vi "Nodos_de_Propiedad_3.vi"() -> ()   [LabVIEW 2016]
panel:
  in  "stop":bool
  out "Boolean":bool
  out "fecha":string
  out "no.muestreo":dbl
  in  "limite superior":dbl
  in  "limite inferior":dbl
  in  "muestras":dbl
  out "temperatura":cluster{dbl, "limite superior":dbl}(graph)
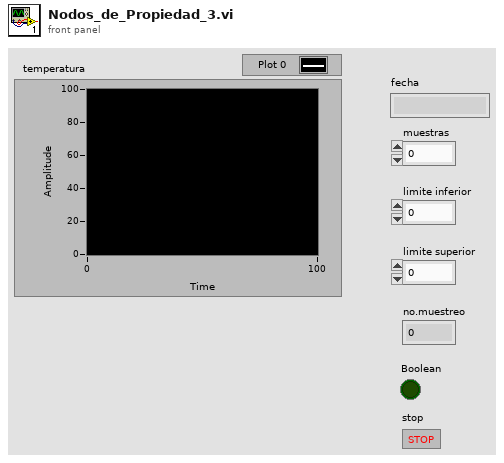
[diagram p1: front panel]
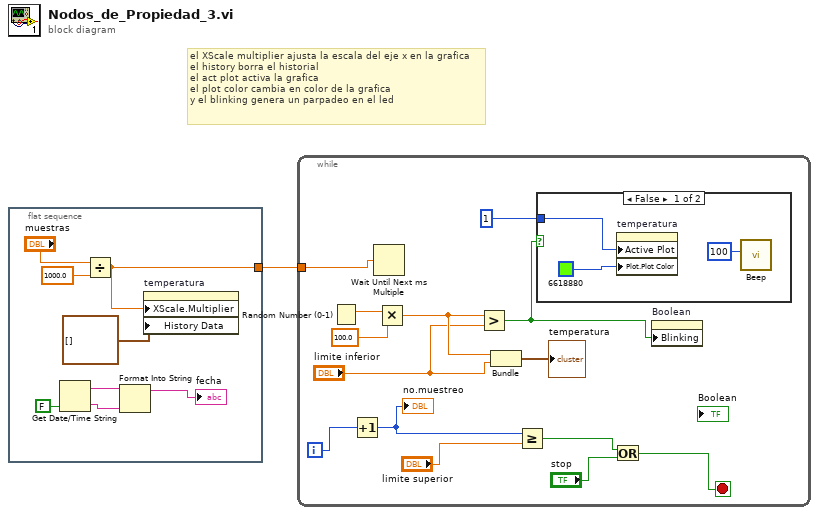
[diagram p0: block diagram]
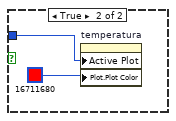
[diagram p2: hidden frame]
diagram:
  # "el XScale multiplier ajusta la escala del eje x en la grafica\nel history borra el historial\nel act plot activa la grafica \nel plot color cambia en color de la grafica\ny el blinking genera un parpadeo en el led"
  n1 = flat-sequence {
    tunnel: [w3] -> w1
    frame #0 {
      n2 = Get Date/Time String(want seconds? (F)=FALSE) -> (date string=w5:string, time string=w6:string)  [unwired: 2 in]
      n3 = Divide(x="muestras", y=1000.0) -> (x/y=w3:dbl)
      n4 = Format Into String(initial string=w5, w6) -> (resulting string=→"fecha":string)  [unwired: 2 in, 1 out]
      n5 = property on="temperatura" class="WFChart (strict)"("XScale.Multiplier"=w3, "History Data"=cluster{dbl, "limite superior":dbl}[] []) -> ()  [unwired: 2 in, 2 out]
    }
  }
  n6 = while {
    tunnel: w1 -> [w23]
    i -> [w20]
    stop <- w15 stop-if-true
    n7 = Random Number (0-1)() -> (number: 0 to 1=w22:dbl)
    n8 = Increment(x=w20) -> (x+1=w19:i32)
    "no.muestreo" <- w19
    n9 = Wait Until Next ms Multiple(millisecond multiple=w23) -> ()  [unwired: 1 out]
    n10 = Multiply(x=w22, y=100.0) -> (x*y=w14:dbl)
    n11 = Greater?(x=w14, y="limite inferior") -> (0:w11:bool)
    n12 = Bundle(w14, "limite inferior"="limite inferior") -> (→"temperatura":cluster{dbl, "limite inferior":dbl})  [unwired: 1 in]
    n13 = Greater Or Equal?(x=w19, y="limite superior") -> (x >= y?=w17:bool)
    n14 = case shown="False" w11 {
      tunnel: 1 -> [w26 w28]
      frame False {
        n15 = property on="temperatura" class="WFChart (strict)"("Active Plot"=w26, "Plot.Plot Color"=u32 6618880) -> ()  [unwired: 2 in, 2 out]
        n16 = call <vilib>:"Beep.vi"("duration (msec)"=u32 100) -> ()  [unwired: 11 in]
      }
      frame True {
        n17 = property on="temperatura" class="WFChart (strict)"("Active Plot"=w28, "Plot.Plot Color"=u32 16711680) -> ()  [unwired: 2 in, 2 out]
      }
    }
    n18 = Or(x=w17, y="stop") -> (x .or. y?=w15:bool)
    n19 = property on="Boolean" class="Bool (strict)"("Blinking"=w11) -> ()  [unwired: 2 in, 2 out]
  }
